vi "DBGetModuleSensors.vi"(7 "Module make":string, 8 "error in (no error)":errorcluster, 9 "Module loc":string, 10 "Module model":string, 11 "db connection in":T1) -> (0 "error out":errorcluster, 1 "sensor chan array":i32[](array[numeric]), 2 "sensor id array":i32[](array[numeric]), 3 "db connection out":T1)   [LabVIEW 2016]
uses:
  <vilib>/addons/database/Connection.llb/Conn ObjectReference.ctl
  <vilib>/addons/database/_DB Variant To Data/Database Variant To Data.xnode
  <vilib>/addons/database/NI_Database_API.lvlib
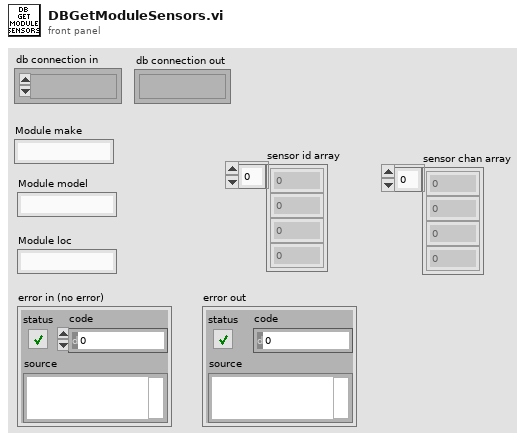
[diagram p1: front panel]
types:
  T1 = typedef "NI_Database_API.lvlib/Conn ObjectReference.ctl" = refnum<k1>
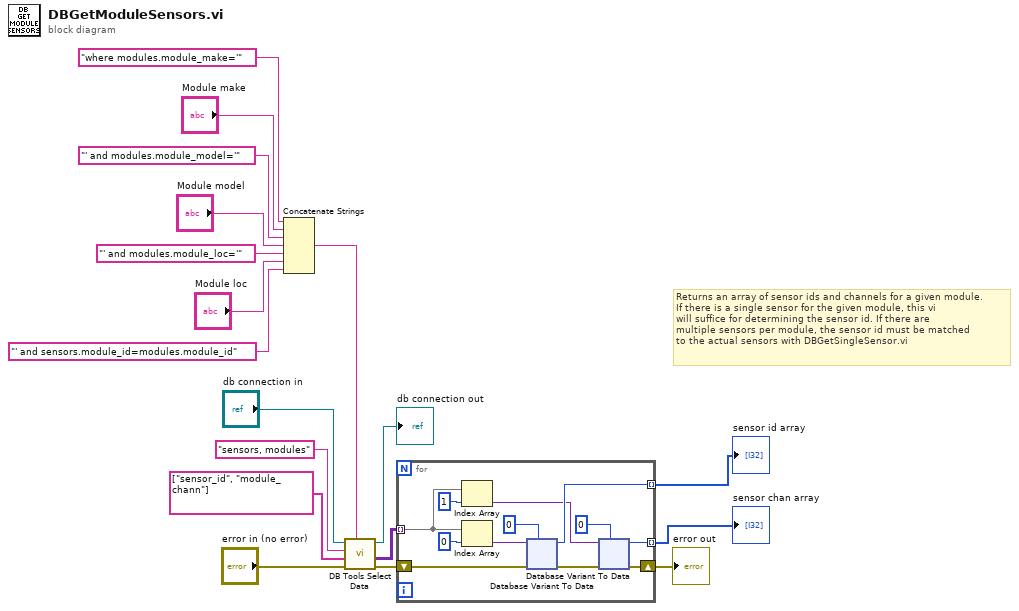
[diagram p0: block diagram]
diagram:
  # "Returns an array of sensor ids and channels for a given module.\nIf there is a single sensor for the given module, this vi\nwill suffice for determining the sensor id. If there are \nmultiple sensors per module, the sensor id must be matched\nto the actual sensors with DBGetSingleSensor.vi"
  n1 = Concatenate Strings("where modules.module_make='" ("string"), "Module make", "' and modules.module_model='" ("string"), "Module model", "' and modules.module_loc='" ("string"), "Module loc", "' and sensors.module_id=modules.module_id" ("string")) -> (w15:string)
  n2 = call <vilib>:"DB Tools Select Data.vi"("condition"=w15, "error in (no error)"="error in (no error)", "columns"=string[] ["sensor_id", "module_chann"], "table"="sensors, modules", "connection reference"="db connection in") -> ("error out"=w17:errorcluster, "data"=w3:variant[][], "connection reference out"=→"db connection out":T1)  [unwired: 1 in]
  n3 = for {
    shift-right: [w19] -> w18
    shift-left: w17 -> [w30]
    tunnel: [w28] -> w1 mode=indexing
    tunnel: w3 -> [w22] mode=indexing
    tunnel: [w21] -> w2 mode=indexing
    n4 = Index Array(array=w22, index=1) -> (element=w24:variant)
    n5 = Index Array(array=w22, index=0) -> (element=w27:variant)
    n6 = xnode "Database Variant To Data"("database variant"=w27, "error in (no error)"=w30, "type"=0) -> ("data"=w28:i32, "error out"=w20:errorcluster)
    n7 = xnode "Database Variant To Data"("database variant"=w24, "error in (no error)"=w20, "type"=0) -> ("data"=w21:i32, "error out"=w19:errorcluster)
  }
  "error out" <- w18
  "sensor id array" <- w1
  "sensor chan array" <- w2
